vi "Variant_ExtractArrayElements.vi"(11 "Array":variant) -> (1 "name":string, 2 "Elements":variant[](array[variant]), 3 "Array dup":variant, 4 "Dimensions":u32[](array[numeric]))   [LabVIEW 2013, in "OpenVariant.lvlib"]
uses:
  OpenVariant.lvlib
  TypeDescriptor/TypeDescriptor_GetPString.vi
  TypeDescriptor/OpenDescriptor.lvlib
  Conversions/OpenConvert.lvlib
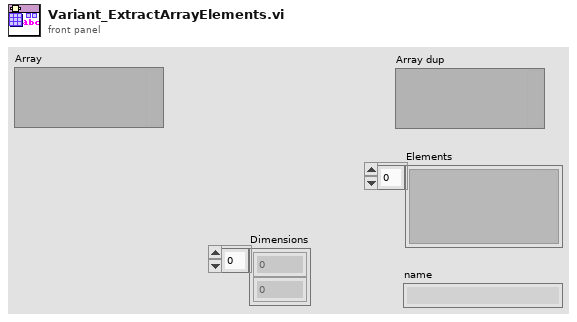
[diagram p1: front panel]
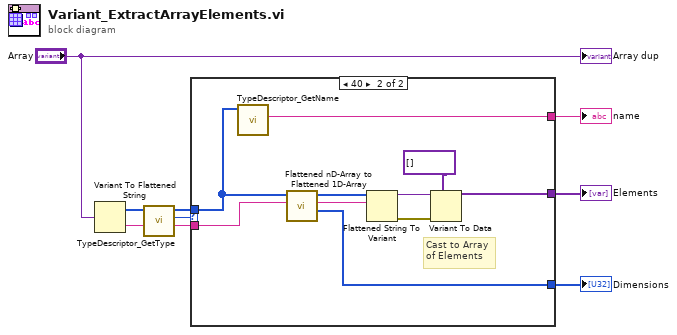
[diagram p0: block diagram]
diagram:
  n1 = Variant To Flattened String(Variant="Array") -> (data string=w6:string, 1:w4:i16[])
  n2 = call "TypeDescriptor_GetType.vi"("type descriptor"=w4) -> ("Type"=w2:u8, "type descriptor dup"=w3:i16[])  [unwired: 9 in]
  n3 = case shown="40" w2 {
    tunnel: [_ w18] -> w8
    tunnel: [_ w17] -> w7
    tunnel: w6 -> [_ w12]
    tunnel: [_ w9] -> w5
    tunnel: w3 -> [_ w13]
    frame Default {
    }
    frame 64 {
      # "Cast to Array\nof Elements"
      n4 = call "TypeDescriptor_GetName.vi"("type descriptor"=w13) -> ("name"=w18:string)  [unwired: 8 in, 2 out]
      n5 = call "Flattened nD-Array to Flattened 1D-Array.vi"("Flattened nD Array"=w12, "nD Array Type Descriptor"=w13) -> ("Original Dimensions"=w9:u32[], "Flattened 1D Array"=w10:string, "1D Array Type Descriptor"=w11:i16[])  [unwired: 7 in]
      n6 = Flattened String To Variant(6:w10, 7:w11) -> (0:w14:errorcluster, 3:w16:variant)  [unwired: 1 in]
      n7 = Variant To Data(error in=w14, type=variant[] [] ("Elements"), Variant=w16) -> (data=w17:variant[])  [unwired: 1 out]
    }
  }
  "Elements" <- w7
  "name" <- w8
  "Dimensions" <- w5
  "Array dup" <- "Array"
